vi "Write Config INI to File.vi"(6 "File Name":string, 7 "File Type":string(combo)=".ini", 8 "Error In":errorcluster, 10 "reference":refnum<vi>, 11 "Path In":path) -> (0 "Error Out":errorcluster, 3 "Path Out":path)   [LabVIEW 2025]
uses:
  <vilib>/Utility/config.llb/Write Key (String).vi
  <vilib>/Utility/config.llb/NI_LVConfig.lvlib
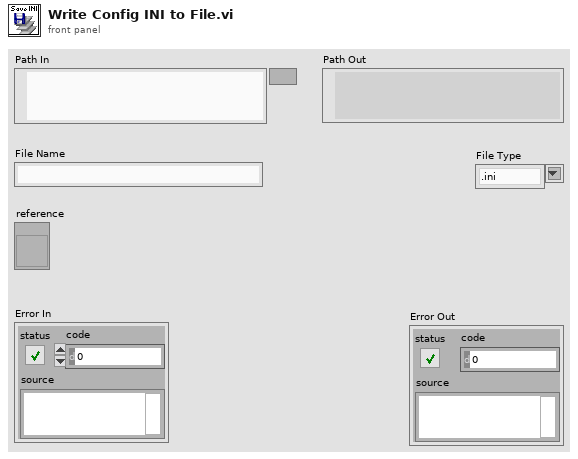
[diagram p1: front panel]
types:
  T1 = typedef "NI_LVConfig.lvlib/Config Data RefNum.ctl" = refnum<k1>
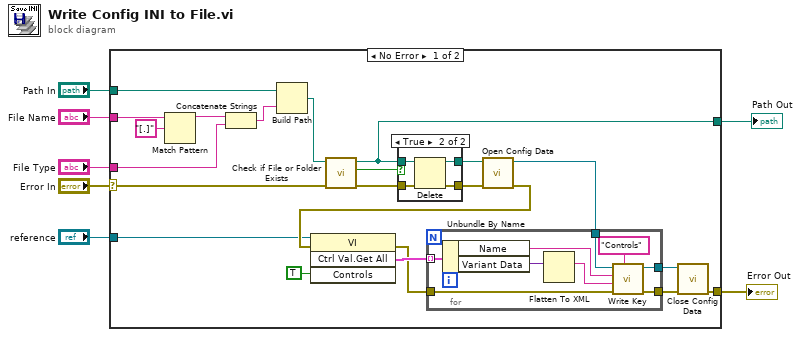
[diagram p0: block diagram]
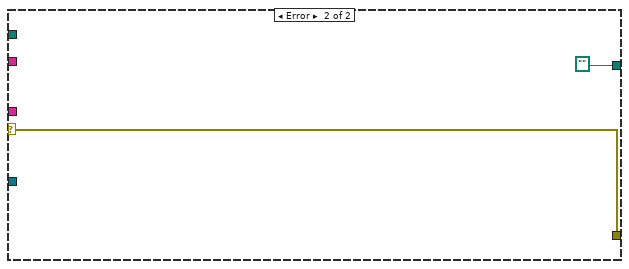
[diagram p3: hidden frame]
diagram:
  n1 = case shown="No Error" "Error In" {
    selector: "Error In" -> [w20 w46]
    tunnel: [w13 w46] -> w2
    tunnel: [w12 path ""] -> w7
    tunnel: "Path In" -> [w9 _]
    tunnel: "File Type" -> [w11 _]
    tunnel: "reference" -> [w10 _]
    tunnel: "File Name" -> [w8 _]
    frame No Error {
      n2 = Match Pattern(string=w8, regular expression="[.]" ("search string")) -> (before substring=w27:string)  [unwired: 1 in, 3 out]
      n3 = Concatenate Strings(w27, w11) -> (w26:string)
      n4 = Build Path(base path=w9, name or relative path=w26) -> (appended path=w21:path)
      n5 = call <vilib>:"Check if File or Folder Exists.vi"("error in (no error)"=w20, "path"=w21) -> ("error out"=w24:errorcluster, "file or folder exists?"=w25:bool, "dup path"=w12:path)  [unwired: 7 in]
      n6 = case shown="True" w25 {
        tunnel: w24 -> [w39 w44]
        tunnel: w12 -> [w40 w43]
        tunnel: [w40 w42] -> w23
        tunnel: [w39 w41] -> w22
        frame False {
        }
        frame True {
          n7 = Delete(path (use dialog)=w43, error in=w44) -> (deleted path=w42:path, error out=w41:errorcluster)  [unwired: 3 in, 1 out]
        }
      }
      n8 = call <vilib>:"Open Config Data.vi"("error in (no error)"=w22, "configuration file path"=w23) -> ("error out"=w17:errorcluster, "refnum"=w18:T1)  [unwired: 1 in, 7 out]
      n9 = invoke class="VI" method="Ctrl Val.Get All"(reference=w10, error in=w17, "Controls"=TRUE) -> (error out=w16:errorcluster, "Get All Control Values Variant"=w19:cluster{"Name":string, "Variant Data":variant}[])  [unwired: 1 in, 2 out]
      n10 = for {
        tunnel: w19 -> [w38] mode=indexing
        tunnel: w18 -> [w35]
        tunnel: w16 -> [w34]
        tunnel: [w31] -> w15
        tunnel: [w30] -> w14
        n11 = Unbundle By Name(w38) -> ("Name"=w33:string, "Variant Data"=w37:variant)
        n12 = Flatten To XML(6:w37) -> (2:w32:string)
        n13 = call-poly <vilib>:"Write Key.vi"("section"="Controls", "error in (no error)"=w34, "value"=w32, "key"=w33, "refnum"=w35) -> ("error out"=w30:errorcluster, "refnum out"=w31:T1)  [unwired: 4 in, 1 out]
      }
      n14 = call <vilib>:"Close Config Data.vi"("error in (no error)"=w14, "refnum"=w15) -> ("error out"=w13:errorcluster)  [unwired: 1 in, 8 out]
    }
    frame Error {
      (unwired) ""
    }
  }
  "Path Out" <- w7
  "Error Out" <- w2
